vi "GV gated pixelclock change.vi"() -> ()   [LabVIEW 2017]
panel:
  out "Gated pixelclock change":bool
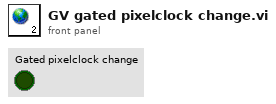
[diagram p1: front panel]
diagram:
